vi "Get.vi"(7 "Entity Manager in":refnum<class "Entity Manager.lvclass">, 11 "Entity in":refnum<class "Entity.lvclass">) -> (1 "error out":errorcluster, 2 "Value":refnum<class "Entity.lvclass">, 3 "Entity":refnum<class "Entity.lvclass">, 5 "Entity Manager":refnum<class "Entity Manager.lvclass">)   [LabVIEW 2020, in "Conditu2.lvlib" / "Columns.lvlib" / "Entity.lvclass"]
uses:
  Entity.lvclass
  Entity/Entity.lvclass
  Entity Manager/Entity Manager.lvclass
  Entity.lvclass/Entity.ctl
  Entity State.ctl
  Entity/Entity.lvclass/Entity.ctl
  ID/ID.lvclass/ID.ctl
  Entity Manager/Entity Manager.lvclass/Entity Manager.ctl
  Entity Manager/Check Unit of Work.vi
  Entity Manager/Get or Register Entity.vi
  Conditu2.lvlib
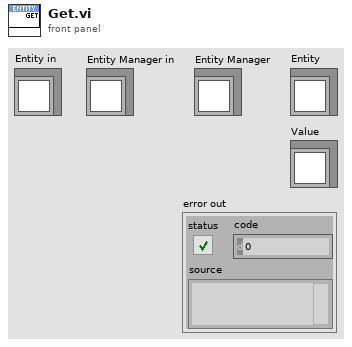
[diagram p1: front panel]
types:
  T1 = typedef "Conditu2.lvlib/Entity State.ctl" = enum16{"New", "Managed", "Detached", "Removed"}
  T2 = typedef "Conditu2.lvlib/Entity ID.ctl" = i64
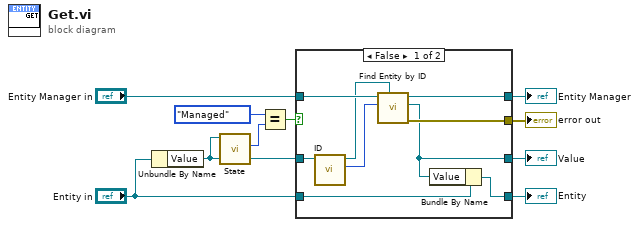
[diagram p0: block diagram]
diagram:
  n1 = Unbundle By Name("Entity in") -> ("Value"=w8:refnum<class "Entity.lvclass">)
  n2 = call "State.vi"("Entity in"=w8) -> ("Entity State"=w10:T1)  [unwired: 10 in]
  n3 = Equal?(x=Entity_State."Managed" ("y"), y=w10) -> (x = y?=w7:bool)
  n4 = case shown="False" w7 {
    tunnel: w8 -> [w18 w22]
    tunnel: [w12 w22] -> w6
    tunnel: "Entity Manager in" -> [w17 w21]
    tunnel: [w16 w21] -> w4
    tunnel: [w19 _] -> w3
    tunnel: "Entity in" -> [w13 w20]
    tunnel: [w11 w20] -> w1
    frame False {
      n5 = call "ID.vi"("Entity in"=w18) -> ("ID"=w15:T2, "Entity out"=w14:refnum<class "Entity.lvclass">)  [unwired: 9 in]
      n6 = call "Find Entity by ID.vi"("Entity Type"=w14, "Entity ID"=w15, "Entity Manager in"=w17) -> ("error out"=w19:errorcluster, "Entity"=w12:refnum<class "Entity.lvclass">, "Entity Manager out"=w16:refnum<class "Entity Manager.lvclass">)  [unwired: 6 in]
      n7 = Bundle By Name(cluster=w13, "Value"=w12) -> (w11:refnum<class "Entity.lvclass">)
    }
    frame True {
    }
  }
  "Value" <- w6
  "Entity Manager" <- w4
  "error out" <- w3
  "Entity" <- w1
